vi "Host Main.vi"() -> ()   [LabVIEW 2015]
doc: "This application launches and executes the Tag Bus Data framework configuration for the specified target alias. This is a simple example of the framework API functions, but may also be a suitable starting point for a Host UI or Thick Client that is running a local version of the framework."
uses:
  <vilib>/NI/Module Execution Interface/Engine Runtime/Execution States.ctl
  <vilib>/NI/Module Execution Interface/Engine Runtime/Fault.ctl
  <vilib>/NI/Tag Bus Module Framework/runtime/error classification.ctl
  <vilib>/userdefined/High Color/nirio_resource_hc.ctl
  <vilib>/NI/Tag Bus Module Framework/FPGA manager/methods.ctl
  <vilib>/NI/Current Value Table/DataTypes/Single_Read.vi
  <vilib>/NI/Current Value Table/Type to Enum.vi
  <vilib>/NI/Current Value Table/DataTypes/Single_Type To Enum.vi
  <vilib>/FPGAPlugInAG/sbRIO-9607/niLvFpga_Open_sbRIO-9607.vi
  <vilib>/rvi/interface/common/dynamic/niFpgaDynamicAddResources.vi
  <vilib>/NI/Current Value Table/FGVs/CVT Globals.vi
  <vilib>/NI/Current Value Table/FGVs/Tag Memory.vi
  <vilib>/NI/Current Value Table/Memory Block.vi
  <vilib>/NI/Current Value Table/DataTypes/Single_Memory Block.vi
  <vilib>/rvi/interface/nirviOpenFPGA/nirviOpenFPGA.xnode
  FPGA Bitfiles/ScaleAndLimit_FPGATarget_BasicFPGATest_5eEjrSJq-IM.lvbitx
  BasicFPGATest.vi
  <vilib>/NI/Module Execution Interface/Engine Runtime/Engine Runtime Interface.lvclass
  <vilib>/NI/DCAF/Tag Editor Core/Framework Configuration Classes/target runtime/PL_Target Runtime.lvclass
  <vilib>/NI/Tag Bus Module Framework/FPGA manager/FPGA manager.lvlib
  <vilib>/NI/Current Value Table/Current Value Table.lvlib
  <vilib>/NI/Tag Bus Module Framework/runtime/TBM module execution interface.lvclass
panel:
  out "Value 3":sgl
  out "Value 2":sgl
  out "Value":sgl
  out "engine status":T4(array[cluster])
  in  "stop":bool
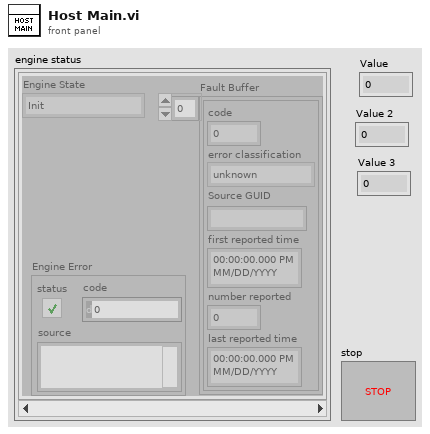
[diagram p1: front panel]
types:
  T1 = typedef "Engine Runtime Interface.lvclass/Execution States.ctl" = enum16{"Init", "Pre-Operational", "Safe-Operational", "Operational", "Stopped"}
  T2 = typedef "Engine Runtime Interface.lvclass/Fault.ctl" = cluster{"code":i32, "error classification":T3, "Source GUID":string, "first reported time":timestamp, "number reported":u32, "last reported time":timestamp}
  T3 = typedef "TBM module execution interface.lvclass/error classification.ctl" = enum16{"unknown", "none", "trivial", "recoverable", "critical"}
  T4 = cluster{"Engine State":T1, "Fault Buffer":T2[], "Engine Error":errorcluster}[]
  T5 = typedef "FPGA manager.lvlib/methods.ctl" = enum16{"initialize bitfile", "cache bitfile", "locate bitfile", "close bitfile", "clear manager"}
  T6 = typedef "nirio_resource_hc.ctl" = tag
  T7 = cluster{"Engine State":T1, "faults":T2[], "Engine Error":errorcluster}
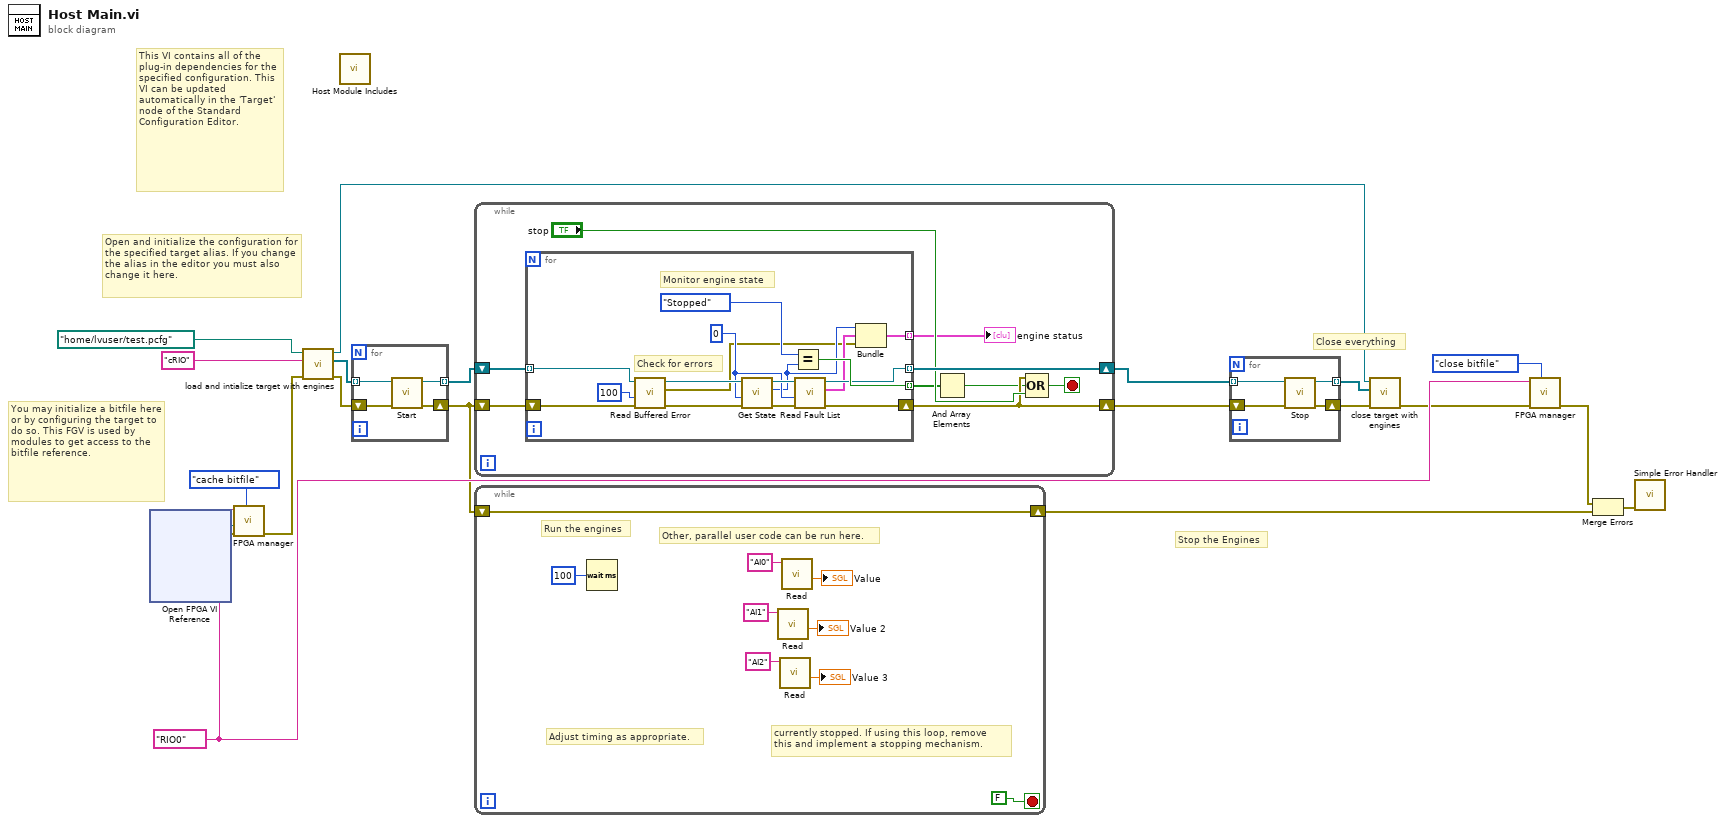
[diagram p0: block diagram]
diagram:
  w10 = T6 "RIO0" ("RIO resource")
  # "You may initialize a bitfile here or by configuring the target to do so. This FGV is used by modules to get access to the bitfile reference."
  # "Open and initialize the configuration for the specified target alias. If you change the alias in the editor you must also change it here."
  # "Close everything"
  # "Stop the Engines"
  # "This VI contains all of the plug-in dependencies for the specified configuration. This VI can be updated automatically in the 'Target' node of the Standard Configuration Editor."
  # "Run the engines"
  n1 = xnode "Open FPGA VI Reference"() -> ("FPGA VI Reference Out"=w3:refnum<k20>, "error out"=w4:errorcluster)  [unwired: 2 in]
  n2 = call <vilib>:"FPGA manager.vi"("action"=methods."cache bitfile", "error in"=w4, "bitfile to cache"=w3, "RIO resource"=w10) -> ("error out"=w11:errorcluster)  [unwired: 5 in, 2 out]
  n3 = call <vilib>:"load and intialize target with engines.vi"("error in"=w11, "target alias"="cRIO", "file path"=path "/home/lvuser/test.pcfg" ("configuration file path")) -> ("error out"=w18:errorcluster, "engine runtime interfaces"=w17:refnum<class "Engine Runtime Interface.lvclass">[], "target runtime"=w14:refnum<class "PL_Target Runtime.lvclass">)  [unwired: 6 in]
  n4 = call "Host Module Includes.vi"() -> ()  [unwired: 12 in]
  n5 = for {
    tunnel: [w25] -> w21 mode=indexing
    tunnel: w17 -> [w22] mode=indexing
    shift-right: [w24] -> w9
    shift-left: w18 -> [w23]
    n6 = call-dynamic "Start.vi"("error in"=w23, "Engine Runtime Interface in"=w22) -> ("error out"=w24:errorcluster, "Engine Runtime Interface out"=w25:refnum<class "Engine Runtime Interface.lvclass">)  [unwired: 8 in]
  }
  n7 = while {
    shift-right: [w32] -> w20
    shift-left: w21 -> [w34]
    shift-right: [w29] -> w19
    shift-left: w9 -> [w33]
    stop <- w30 stop-if-true
    n8 = for {
      tunnel: w34 -> [w50] mode=indexing
      tunnel: [w41] -> w32 mode=indexing
      tunnel: [w45] -> w27 mode=indexing
      shift-right: [w40] -> w29
      shift-left: w33 -> [w49]
      tunnel: [w35] -> w28 mode=indexing
      w39 = 0 ("timeout (-1)")
      # "Monitor engine state"
      # "Check for errors"
      n9 = call-dynamic "Read Buffered Error.vi"("error in"=w49, "timeout in ms (0)"=100, "Engine Runtime Interface in"=w50) -> ("error out"=w47:errorcluster, "Engine Error"=w36:errorcluster, "Engine Runtime Interface out"=w48:refnum<class "Engine Runtime Interface.lvclass">)  [unwired: 6 in]
      n10 = call-dynamic "Get State.vi"("error in"=w47, "timeout (-1)"=w39, "Engine Runtime Interface in"=w48) -> ("error out"=w43:errorcluster, "Engine State"=w38:T1, "Engine Runtime Interface out"=w42:refnum<class "Engine Runtime Interface.lvclass">)  [unwired: 6 in]
      n11 = Equal?(x=Execution_States."Stopped" ("Engine State"), y=w38) -> (x = y?=w45:bool)
      n12 = call-dynamic "Read Fault List.vi"("error in"=w43, "timeout (-1)"=w39, "Engine Runtime Interface in"=w42) -> ("error out"=w40:errorcluster, "faults"=w37:T2[], "Engine Runtime Interface out"=w41:refnum<class "Engine Runtime Interface.lvclass">)  [unwired: 6 in]
      n13 = Bundle("Engine State"=w38, "faults"=w37, "Engine Error"=w36) -> (w35:T7)  [unwired: 1 in]
    }
    "engine status" <- w28
    n14 = And Array Elements(Boolean array=w27) -> (logical AND=w26:bool)
    n15 = Compound Arithmetic op=OR(w29, w26, "stop") -> (w30:bool)
  }
  n16 = while {
    shift-right: [w57] -> w8
    shift-left: w9 -> [w57]
    stop <- FALSE stop-if-true
    # "currently stopped. If using this loop, remove \nthis and implement a stopping mechanism."
    # "Adjust timing as appropriate."
    # "Other, parallel user code can be run here."
    n17 = Wait (ms)(milliseconds to wait=u32 100) -> ()  [unwired: 1 out]
    n18 = call-poly <vilib>:"Read.vi"("Tag Name"="AI1") -> ("Value"=→"Value 2":sgl)  [unwired: 9 in, 1 out]
    n19 = call-poly <vilib>:"Read.vi"("Tag Name"="AI2") -> ("Value"=→"Value 3":sgl)  [unwired: 9 in, 1 out]
    n20 = call-poly <vilib>:"Read.vi"("Tag Name"="AI0") -> ("Value"=→"Value":sgl)  [unwired: 9 in, 1 out]
  }
  n21 = for {
    tunnel: w20 -> [w63] mode=indexing
    shift-right: [w60] -> w13
    shift-left: w19 -> [w62]
    tunnel: [w61] -> w15 mode=indexing
    n22 = call-dynamic "Stop.vi"("error in"=w62, "Engine Runtime Interface in"=w63) -> ("error out"=w60:errorcluster, "Engine Runtime Interface out"=w61:refnum<class "Engine Runtime Interface.lvclass">)  [unwired: 8 in]
  }
  n23 = call <vilib>:"close target with engines.vi"("error in"=w13, "Engine Runtime Interfaces"=w15, "Target Runtime"=w14) -> ("error out"=w7:errorcluster)  [unwired: 8 in]
  n24 = call <vilib>:"FPGA manager.vi"("action"=methods."close bitfile", "error in"=w7, "RIO resource"=w10) -> ("error out"=w6:errorcluster)  [unwired: 6 in, 2 out]
  n25 = Merge Errors(w6, w8) -> (w5:errorcluster)
  n26 = call <vilib>:"Simple Error Handler.vi"("error in (no error)"=w5) -> ()  [unwired: 4 in, 5 out]
